vi "FindClosestPointArray.vi"(8 "Y":sgl, 9 "X":sgl, 11 "Particle Measurements (Pixels)":sgl[][](array[numeric]) format="%.2f") -> (2 "ShortestDistanceIndex":i32, 3 "ShortestDistance":sgl)   [LabVIEW 2019]
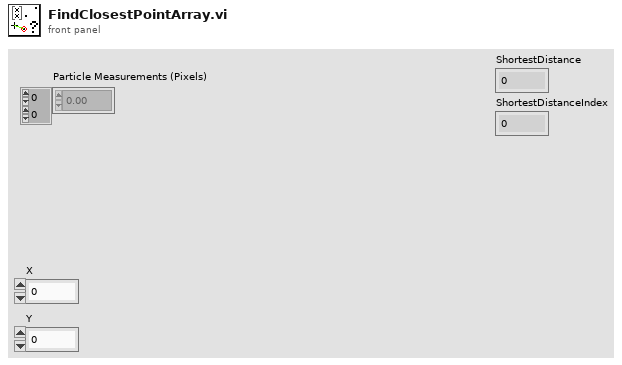
[diagram p1: front panel]
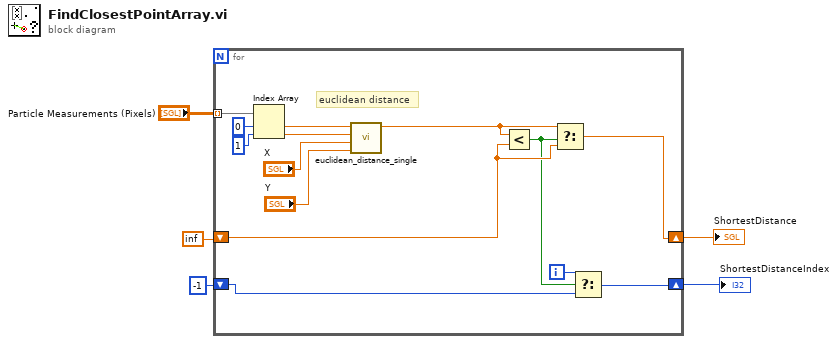
[diagram p0: block diagram]
diagram:
  n1 = for {
    shift-right: [w18] -> w3
    shift-left: inf -> [w19]
    shift-right: [w17] -> w2
    shift-left: -1 -> [w14]
    tunnel: "Particle Measurements (Pixels)" -> [w10] mode=indexing
    i -> [w15]
    # "euclidean distance"
    n2 = Index Array(array=w10, index #1=0 ("index"), index #2=1 ("index")) -> (element #1=w8:sgl, element #2=w6:sgl)
    n3 = call "euclidean_distance_single.vi"("Point 2 Y"="Y", "Point 2 X"="X", "Point 1 Y"=w6, "Point 1 X"=w8) -> ("Distance"=w11:sgl)  [unwired: 7 in]
    n4 = Less?(x=w11, y=w19) -> (x < y?=w16:bool)
    n5 = Select(t=w11, s=w16, f=w19) -> (s? t:f=w18:dbl)
    n6 = Select(t=w15, s=w16, f=w14) -> (s? t:f=w17:i32)
  }
  "ShortestDistance" <- w3
  "ShortestDistanceIndex" <- w2
